vi "graph sine array.vi"() -> ()   [LabVIEW 2016]
uses:
  <vilib>/Utility/file.llb/Write Delimited Spreadsheet (DBL).vi
panel:
  out "Cos Waveform Array":dbl[](array[numeric])
  out "Waveform Graph":dbl[][](graph)
  out "Sine Waveform Array":dbl[](array[numeric])
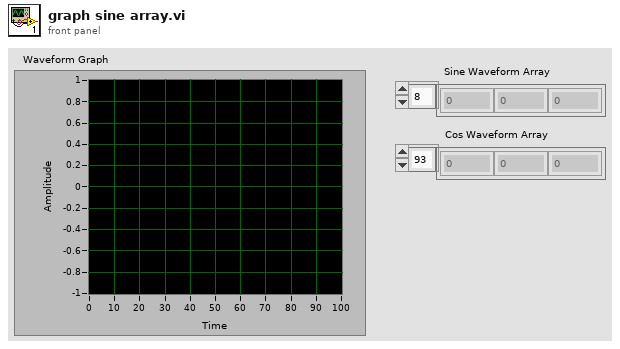
[diagram p1: front panel]
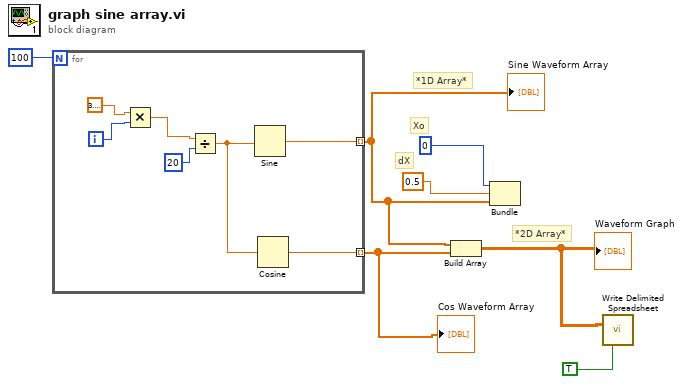
[diagram p0: block diagram]
diagram:
  # "*1D Array*"
  # "*2D Array*"
  # "dX"
  # "Xo"
  n1 = for {
    N: 100 -> [_]
    tunnel: [w10] -> w4 mode=indexing
    tunnel: [w8] -> w3 mode=indexing
    i -> [w13]
    n2 = Multiply(x=3.141592653589793, y=w13) -> (x*y=w12:dbl)
    n3 = Divide(x=w12, y=20) -> (x/y=w9:dbl)
    n4 = Sine(x=w9) -> (sin(x)=w10:dbl)
    n5 = Cosine(x=w9) -> (cos(x)=w8:dbl)
  }
  "Sine Waveform Array" <- w4
  "Cos Waveform Array" <- w3
  n6 = Build Array(w4, w3) -> (w2:dbl[][])
  "Waveform Graph" <- w2
  n7 = Bundle(0, 0.5, w4) -> ()  [unwired: 1 in, 1 out]
  n8 = call-poly <vilib>:"Write Delimited Spreadsheet.vi"("2D data"=w2, "transpose? (no:F)"=TRUE) -> ()  [unwired: 12 in, 2 out]
